vi "Vision_Test2.vi"() -> ()   [LabVIEW 2011]
panel:
  out "Ready":bool
  out "Elevation Angle":dbl
  out "Shortest Dist To Rect Center":dbl
  in  "Threshold Range":cluster{"Lower value":sgl, "Upper value":sgl}={"Lower value"=240.0, "Upper value"=255.0}
  in  "Milsec Wait":u32=5000
  in  "Take Pics":bool
  out "Image 2":T1(plugin-control)
  out "Image 1":T1(plugin-control)
  out "Binary Image 2":T1(plugin-control)
  out "Binary Image 1":T1(plugin-control)
  out "Processed Image":T1(plugin-control)
  out "Offset Angle From Perpendicular":dbl
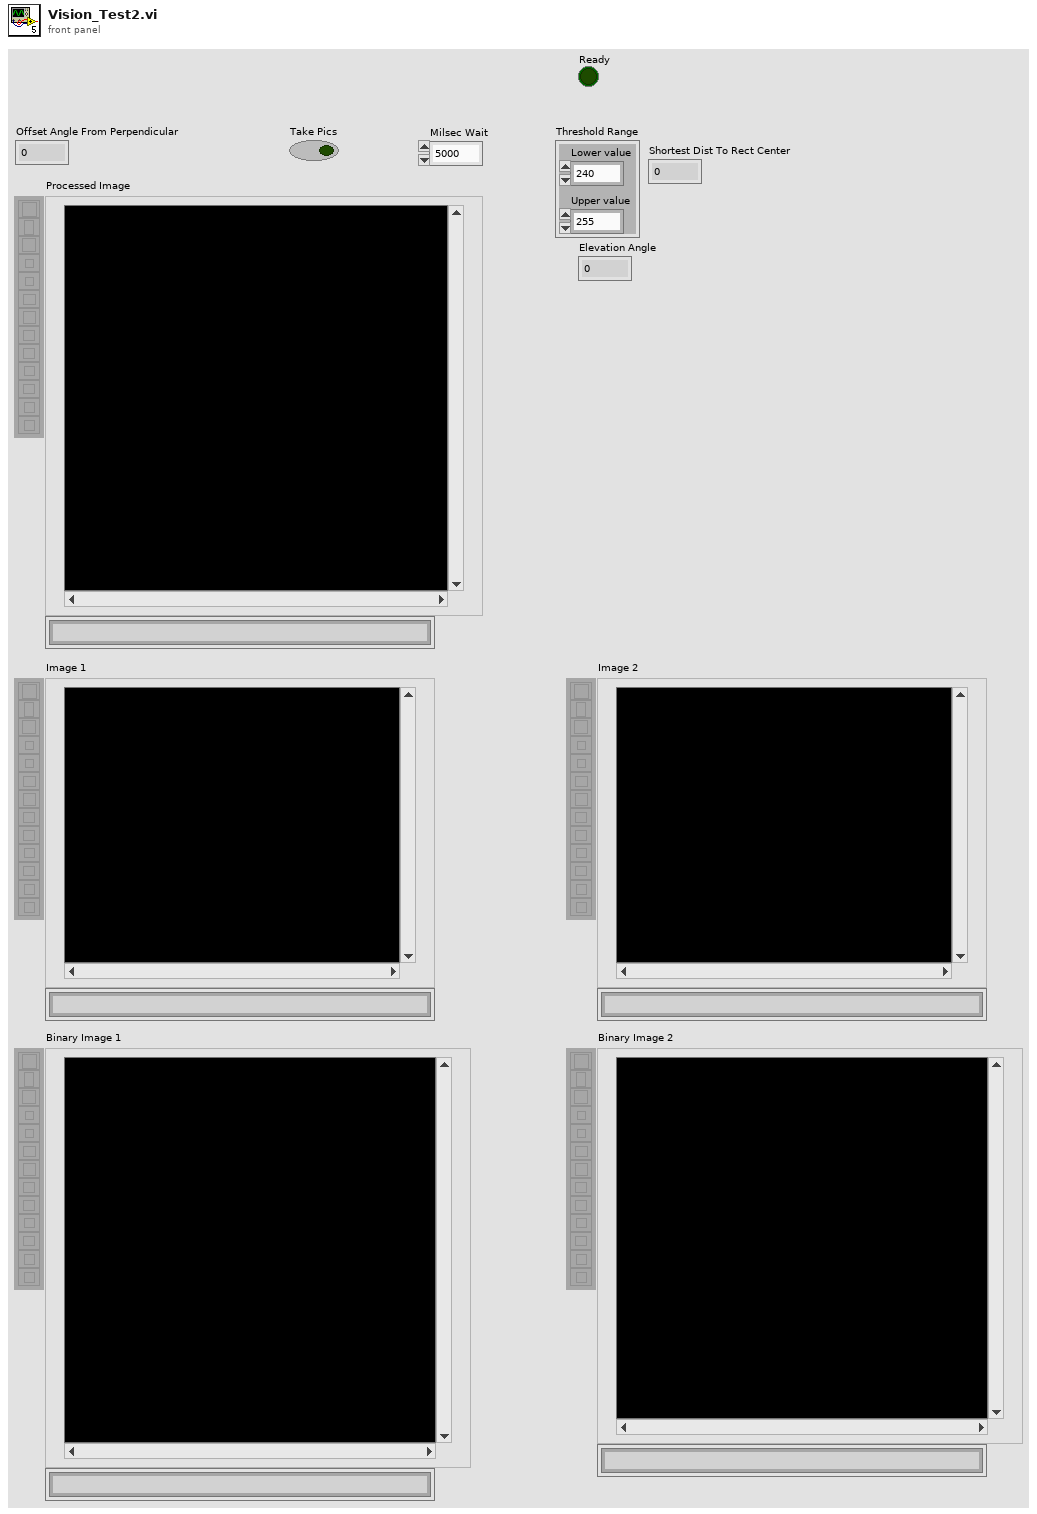
[diagram p1: front panel]
types:
  T1 = typedef "IMAQ Image.ctl" = refnum<image>
  T2 = typedef "WPI_CameraDevRef.ctl" = cluster{"Camera Address":string, "CameraStatus":errorcluster, "Acquire Image Notifier":refnum<notifier>}
  T3 = cluster{"Image_Dsts_Out[0]":T1, "Image_Dsts_Out[1]":T1, "Image_Dsts_Out[2]":T1, "Image_Dsts_Out[3]":T1, "Image_Dsts_Out[4]":T1, "Image_Dsts_Out[5]":T1, "Image_Dsts_Out[6]":T1, "Image_Dsts_Out[7]":T1, "Image_Dsts_Out[8]":T1}
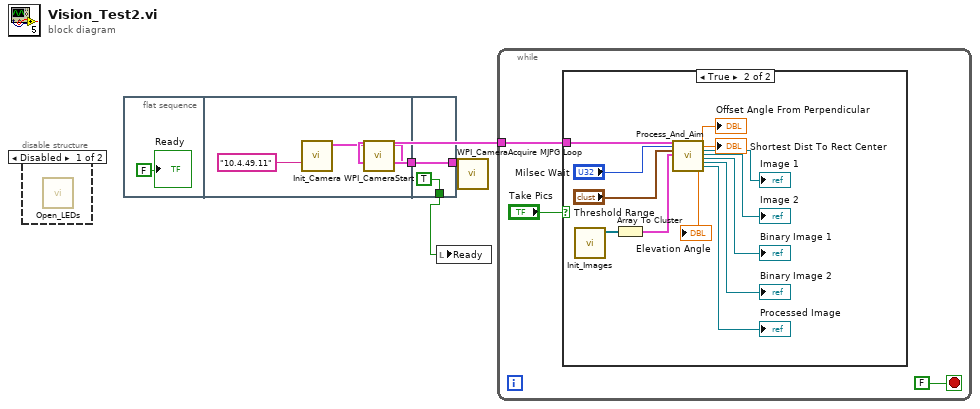
[diagram p0: block diagram]
diagram:
  n1 = disable-structure shown="Disabled" {
    frame Disabled {
      n2 = call "Open_LEDs.vi"() -> ()  [unwired: 11 in, 1 out]
    }
    frame Enabled {
    }
  }
  n3 = flat-sequence {
    tunnel: [w7] -> w2
    tunnel: [w9] -> w3
    tunnel: w2 -> [w9]
    tunnel: [TRUE] -> w1
    frame #0 {
      "Ready" <- FALSE
    }
    frame #1 {
      n4 = call "Init_Camera.vi"("Camera IP"="10.4.49.11") -> ("CameraDevRef Out"=w5:T2)  [unwired: 10 in]
      n5 = call <vilib>:"WPI_CameraStart.vi"("CameraDevRef"=w5) -> ("CameraDevRef Out"=w7:T2)  [unwired: 9 in, 1 out]
    }
    frame #2 {
    }
  }
  n6 = local write "Ready"(w1) -> ()
  n7 = call <vilib>:"WPI_CameraAcquire MJPG Loop.vi"("CameraDevRef"=w3) -> ()  [unwired: 11 in]
  n8 = while {
    tunnel: w3 -> [w12]
    stop <- FALSE stop-if-true
    n9 = case shown="True" "Take Pics" {
      tunnel: w12 -> [_ w25]
      frame False {
      }
      frame True {
        n10 = call "Init_Images.vi"() -> ("Image_Dsts_Out"=w16:T1[])  [unwired: 11 in]
        n11 = Array To Cluster(array=w16) -> (cluster=w15:T3)
        n12 = call "Process_And_Aim.vi"("CameraDevRef"=w25, "Milsec Wait"="Milsec Wait", "Threshold Range"="Threshold Range", "Image Dsts Clust"=w15) -> ("Offset Angle From Perpendicular"=→"Offset Angle From Perpendicular":dbl, "Shortest Dist To Rect Center"=→"Shortest Dist To Rect Center":dbl, "Image 1 Out"=→"Image 1":T1, "Image 2 Out"=→"Image 2":T1, "Binary 1 Out"=→"Binary Image 1":T1, "Binary 2 Out"=→"Binary Image 2":T1, "Processed Image Out"=→"Processed Image":T1, "Elevation Angle"=→"Elevation Angle":dbl)  [unwired: 16 in]
      }
    }
  }
